vi "Figure Gen.vi"() -> ()   [LabVIEW 2016]
panel:
  out "M/G v Temp":T1(graph)
  out "M/G v Temp Normalized":T1(graph)
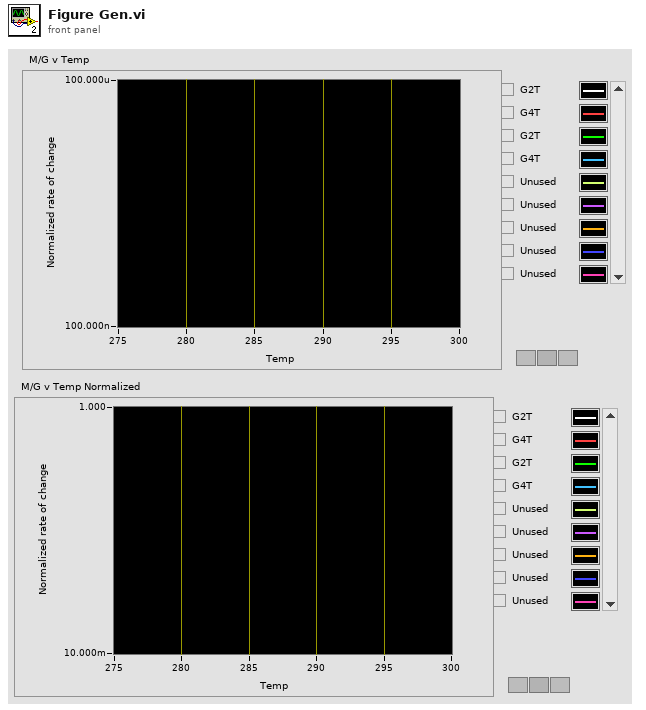
[diagram p1: front panel]
types:
  T1 = cluster{"Data":dbl[], "Best Exponential Fit":dbl[]}[]
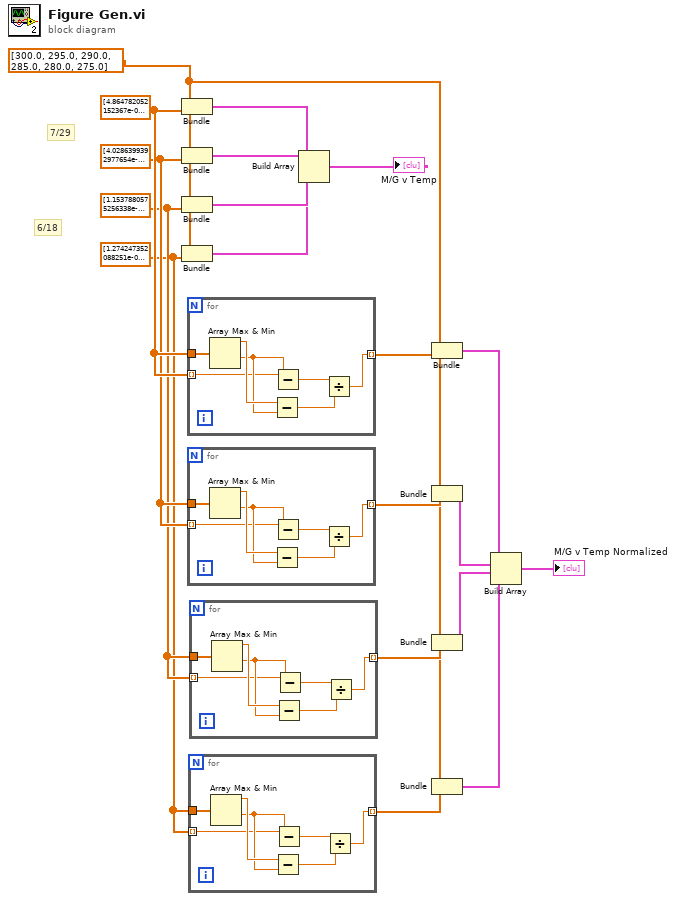
[diagram p0: block diagram]
diagram:
  w10 = dbl[] [1.1537880575256338e-05, 4.22826060820674e-06, 2.3653742417541264e-06, 1.3028566769234502e-06, 7.890287594859811e-07, 4.7153090154693677e-07] ("M2T")
  w9 = dbl[] [1.274247352088251e-05, 4.55980820011919e-06, 2.5020592499196788e-06, 1.3489355716779094e-06, 7.925451445036797e-07, 4.908004729274311e-07] ("M4T")
  w2 = dbl[] [300.0, 295.0, 290.0, 285.0, 280.0, 275.0]
  w11 = dbl[] [4.0286399392977654e-05, 1.1934183863055551e-05, 5.895450541703924e-06, 3.85186272225402e-06, 2.6126636167088024e-06, 1.8906421875696023e-06] ("x/y 2")
  w12 = dbl[] [4.864782052152367e-05, 1.4394380255731984e-05, 7.063298030319999e-06, 4.797818894900328e-06, 3.0858711624502367e-06, 2.185253068975472e-06] ("x/y")
  # "7/29"
  # "6/18"
  n1 = Bundle(w2, "x/y"=w12) -> (w19:cluster{dbl[], "x/y":dbl[]})  [unwired: 1 in]
  n2 = Bundle(w2, "x/y 2"=w11) -> (w18:cluster{dbl[], "x/y 2":dbl[]})  [unwired: 1 in]
  n3 = Bundle(w2, "M2T"=w10) -> (w17:cluster{dbl[], "M2T":dbl[]})  [unwired: 1 in]
  n4 = Bundle(w2, "M4T"=w9) -> (w16:cluster{dbl[], "M4T":dbl[]})  [unwired: 1 in]
  n5 = for {
    tunnel: [w25] -> w14 mode=indexing
    tunnel: w12 -> [w24]
    tunnel: w12 -> [w21] mode=indexing
    n6 = Array Max & Min(array=w24) -> (max value=w23:dbl, min value=w22:dbl)  [unwired: 2 out]
    n7 = Subtract(x=w23, y=w22) -> (x-y=w20:dbl)
    n8 = Subtract(x=w21, y=w22) -> (x-y=w26:dbl)
    n9 = Divide(x=w26, y=w20) -> (x/y=w25:dbl)
  }
  n10 = for {
    tunnel: [w32] -> w6 mode=indexing
    tunnel: w11 -> [w31]
    tunnel: w11 -> [w28] mode=indexing
    n11 = Array Max & Min(array=w31) -> (max value=w30:dbl, min value=w29:dbl)  [unwired: 2 out]
    n12 = Subtract(x=w30, y=w29) -> (x-y=w27:dbl)
    n13 = Subtract(x=w28, y=w29) -> (x-y=w33:dbl)
    n14 = Divide(x=w33, y=w27) -> (x/y=w32:dbl)
  }
  n15 = for {
    tunnel: [w39] -> w8 mode=indexing
    tunnel: w9 -> [w38]
    tunnel: w9 -> [w35] mode=indexing
    n16 = Array Max & Min(array=w38) -> (max value=w37:dbl, min value=w36:dbl)  [unwired: 2 out]
    n17 = Subtract(x=w37, y=w36) -> (x-y=w34:dbl)
    n18 = Subtract(x=w35, y=w36) -> (x-y=w40:dbl)
    n19 = Divide(x=w40, y=w34) -> (x/y=w39:dbl)
  }
  n20 = for {
    tunnel: [w46] -> w7 mode=indexing
    tunnel: w10 -> [w45]
    tunnel: w10 -> [w42] mode=indexing
    n21 = Array Max & Min(array=w45) -> (max value=w44:dbl, min value=w43:dbl)  [unwired: 2 out]
    n22 = Subtract(x=w44, y=w43) -> (x-y=w41:dbl)
    n23 = Subtract(x=w42, y=w43) -> (x-y=w47:dbl)
    n24 = Divide(x=w47, y=w41) -> (x/y=w46:dbl)
  }
  n25 = Build Array(w19, w18, w17, w16) -> (→"M/G v Temp":cluster{dbl[], "M4T":dbl[]}[])
  n26 = Bundle(w2, w14) -> (w13:cluster{dbl[], dbl[]})  [unwired: 1 in]
  n27 = Bundle(w2, w6) -> (w5:cluster{dbl[], dbl[]})  [unwired: 1 in]
  n28 = Bundle(w2, w7) -> (w4:cluster{dbl[], dbl[]})  [unwired: 1 in]
  n29 = Bundle(w2, w8) -> (w3:cluster{dbl[], dbl[]})  [unwired: 1 in]
  n30 = Build Array(w13, w5, w4, w3) -> (→"M/G v Temp Normalized":cluster{dbl[], dbl[]}[])
